vi "Write timeouts.vi"(8 "error in (no error)":errorcluster, 10 "SP timeouts":T1={"reconn_timeout"=3000, "read_timeout"=1000, "N attempt max"=3, "t_reset_TTL"=120000, "period"=100} {"read_timeout" min=1 max=5 step=1; "t_reset_TTL" min=10 max=100000 step=1; "period" min=10 max=100000 step=1; "N attempt max" min=10 max=240000 step=1; "reconn_timeout" min=10 max=240000 step=1}, 11 "SP in":refnum<class "Save messages PGserver.lvclass">) -> (0 "error out":errorcluster, 3 "SP out":refnum<class "Save messages PGserver.lvclass">)   [LabVIEW 2019, in "Save messages PGserver.lvclass"]
uses:
  Save messages PGserver.lvclass
  ctl/Save_prog_timeouts.ctl
  Save messages PGserver.lvclass/Save messages PGserver.ctl
  PostgreSQL.lvlib
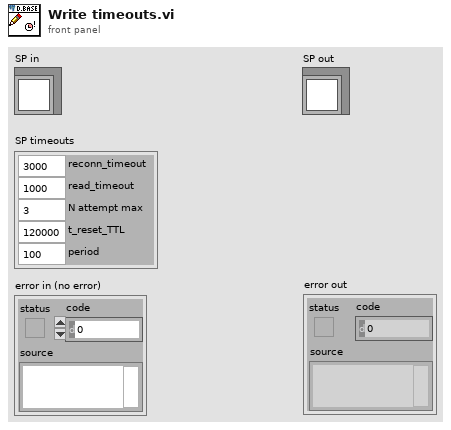
[diagram p1: front panel]
types:
  T1 = typedef "PostgreSQL.lvlib/Save_prog_timeouts.ctl" = cluster{"reconn_timeout":i32, "read_timeout":i32, "N attempt max":i32, "t_reset_TTL":i32, "period":i32}
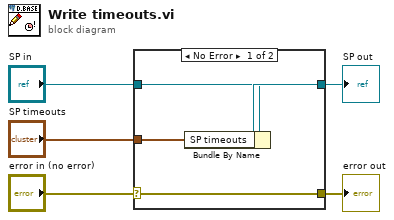
[diagram p0: block diagram]
diagram:
  n1 = case shown="No Error" "error in (no error)" {
    selector: "error in (no error)" -> [w9 w10]
    tunnel: [w9 w10] -> w4
    tunnel: [w7 w11] -> w2
    tunnel: "SP in" -> [w6 w11]
    tunnel: "SP timeouts" -> [w8 _]
    frame No Error {
      n2 = Bundle By Name(cluster=w6, "SP timeouts"=w8) -> (w7:refnum<class "Save messages PGserver.lvclass">)
    }
    frame Error {
    }
  }
  "error out" <- w4
  "SP out" <- w2
